vi "Validate_Do.vi"(8 "error in (no error)":errorcluster, 11 "Action in":refnum<class "Project Action.lvclass">) -> (0 "error out":errorcluster, 1 "Valid?":bool, 3 "Action out":refnum<class "Project Action.lvclass">)   [LabVIEW 2019, in "ProjectBuilder.lvlib" / "Project Action.lvclass"]
doc: "Override to validate the class.\n\nThe default implementation does nothing but return 'Success?'=True."
uses:
  Class/Project Action/Project Action.lvclass
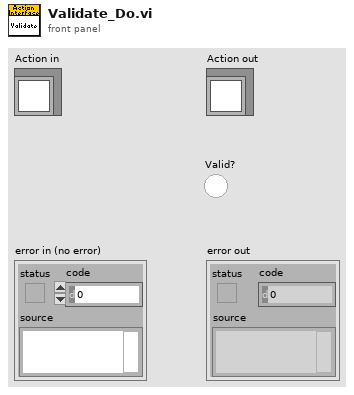
[diagram p1: front panel]
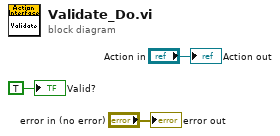
[diagram p0: block diagram]
diagram:
  "error out" <- "error in (no error)"
  "Action out" <- "Action in"
  "Valid?" <- TRUE
